vi "LVClass_WavefrontCorrector ctor.vi"(0 "WavefrontCorrector (const)":refnum<class "WavefrontCorrector.lvclass">, 5 "PathToWavefrontCorrectorSetupFile":path, 7 "init_state_from_config_file":bool, 11 "error in (no error)":errorcluster) -> (4 "WavefrontCorrector (new)":refnum<class "WavefrontCorrector.lvclass">, 15 "error out":errorcluster)   [LabVIEW 2020, in "WavefrontCorrector.lvclass"]
doc: "WavefrontCorrector constructor.\n\n--------------------------------------------------------------------------------\n\n<B>correctorIn </B> : Constant Pointer to WavefrontCorrector object.\n<B>correctorOut </B> : Constant Pointer to WavefrontCorrector object.\n<B>config_file_path </B> : Absolute path to Wavefront corrector configuration file.\n<B>ErrorIn </B> : Error\n<B>ErrorOut </B> : Error\n\n--------------------------------------------------------------------------------"
uses:
  WavefrontCorrector.lvclass
  WavefrontCorrectorSet.lvclass
  Wavefront Corrector states - ONE.ctl
  WavefrontCorrector.lvclass/WavefrontCorrector.ctl
  Handle creation.ctl
  LVClass_WavefrontCorrectorSet Read AllWavefrontCorrectorParametersProperties.vi
  LVClass_WavefrontCorrectorSet Read AllValueSetAndGet.vi
  LVClass_WavefrontCorrectorSet Read AllValueGet.vi
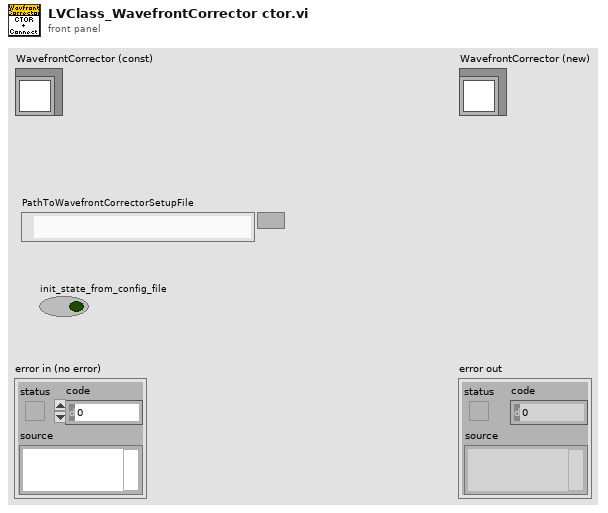
[diagram p1: front panel]
types:
  T1 = typedef "Wavefront Corrector states - ONE.ctl" = cluster{"Max":sgl, "Min":sgl, "Validity":enum16{"valid", "fixed", "invalid"}, "Fixed_Position":sgl}
  T2 = typedef "Handle creation.ctl" = enum16{"By ctor", "By write function"}
  T3 = typedef "WavefrontCorrectorSpecifications.ctl" = cluster{"Mirror name":string, "Plugin name":string, "Serial number":string, "Revision":string, "Number of commands":i32, "Sleep after command apply (ms)":i32, "Has internal memory ?":bool}
  T4 = typedef "ParameterID.ctl" = cluster{"Name":string, "ConnectionParameter?":bool, "Type":T5, "Authorization":T6, "OnFlyAuthorization":T7, "StringValue":string, "Value":dbl, "Min":dbl, "Max":dbl, "BooleanValue":bool, "StringParameterList":string[]}
  T5 = typedef "CameraParameters_Type.ctl" = enum16{"Integer", "Real", "String", "Boolean"}
  T6 = typedef "CameraParameters_Authorization.ctl" = enum16{"Disable", "Gettable", "Settable - Gettable"}
  T7 = typedef "CameraParameters_OnFlyAuthorization.ctl" = enum16{"None", "Gettable", "Settable", "Settable - Gettable"}
  T8 = typedef "CameraParametersSetup.ctl" = cluster{"Name":string, "Type":T5, "Value":dbl, "BooleanValue":bool, "StringValue":string, "ConnectionParameter":bool}
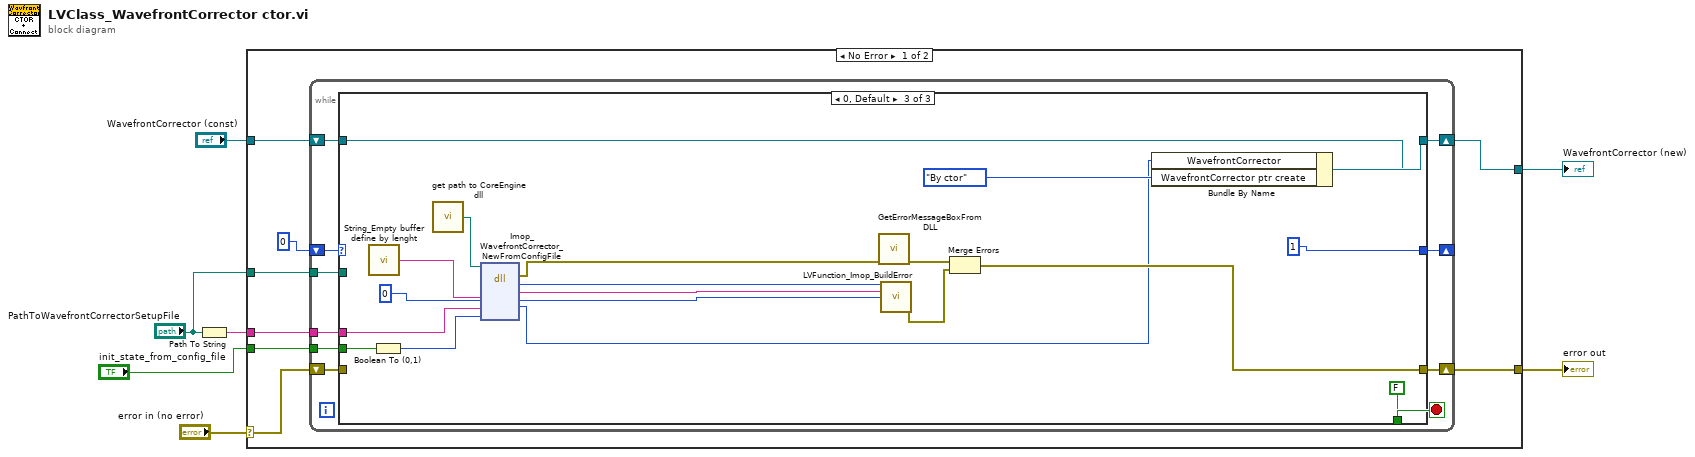
[diagram p0: block diagram]
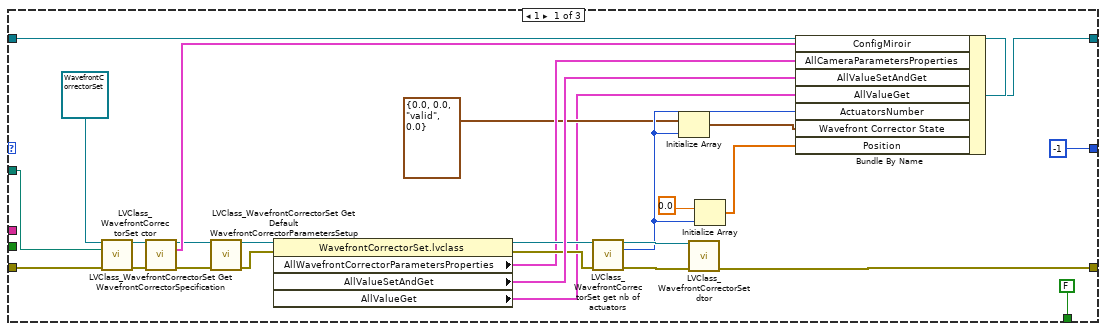
[diagram p2: hidden frame]
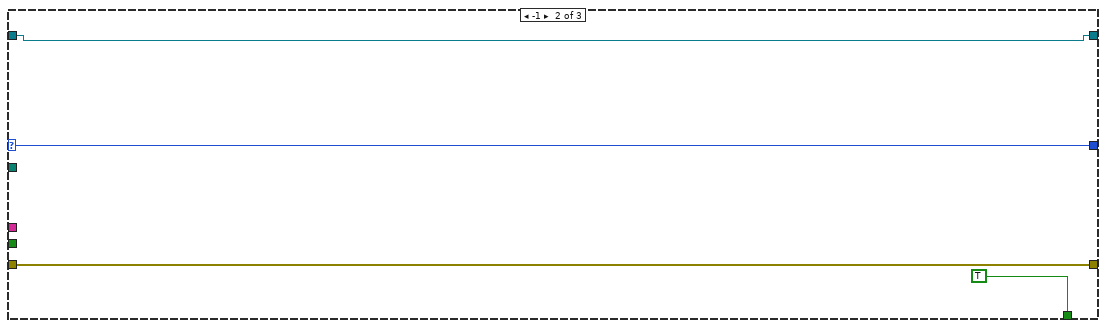
[diagram p3: hidden frame]
diagram:
  n1 = Path To String(path="PathToWavefrontCorrectorSetupFile") -> (string=w7:string)
  n2 = case shown="No Error" "error in (no error)" {
    selector: "error in (no error)" -> [w10 w76]
    tunnel: [w9 w76] -> w4
    tunnel: [w14 w75] -> w3
    tunnel: "WavefrontCorrector (const)" -> [w15 w75]
    tunnel: w7 -> [w13 _]
    tunnel: "PathToWavefrontCorrectorSetupFile" -> [w11 _]
    tunnel: "init_state_from_config_file" -> [w8 _]
    frame No Error {
      n3 = while {
        tunnel: w13 -> [w24]
        shift-right: [w22] -> _
        shift-left: 0 -> [w23]
        tunnel: w11 -> [w21]
        shift-right: [w18] -> w9
        shift-left: w10 -> [w19]
        shift-right: [w25] -> w14
        shift-left: w15 -> [w20]
        tunnel: w8 -> [w16]
        stop <- w17 stop-if-true
        n4 = case shown="0, Default" w23 {
          selector: w23 -> [_ w56 _]
          tunnel: [w40 w53 w68] -> w25
          tunnel: [w41 w55 w65] -> w18
          tunnel: w24 -> [_ _ w64]
          tunnel: [-1 w56 1] -> w22
          tunnel: w21 -> [w50 _ _]
          tunnel: w20 -> [w49 w53 w61]
          tunnel: w19 -> [w46 w55 _]
          tunnel: [FALSE TRUE FALSE] -> w17
          tunnel: w16 -> [_ _ w59]
          frame 1 {
            n5 = call "LVClass_WavefrontCorrectorSet ctor.vi"("WavefrontCorrectorSet (const)"=refnum<class "WavefrontCorrectorSet.lvclass"> refnum ("WavefrontCorrectorSet.lvclass"), "PathToWavefrontCorrectorSetupFile"=w50, "error in (no error)"=w46) -> ("WavefrontCorrectorSet (new)"=w52:refnum<class "WavefrontCorrectorSet.lvclass">, "error out"=w47:errorcluster)  [unwired: 11 in]
            n6 = call "LVClass_WavefrontCorrectorSet Get WavefrontCorrectorSpecification.vi"("WavefrontCorrectorSet in"=w52, "error in (no error)"=w47) -> ("WavefrontCorrectorSet out"=w34:refnum<class "WavefrontCorrectorSet.lvclass">, "ConfigMiroir"=w48:T3, "error out"=w35:errorcluster)  [unwired: 11 in]
            n7 = call "LVClass_WavefrontCorrectorSet Get Default WavefrontCorrectorParametersSetup.vi"("WavefrontCorrectorSet in"=w34, "error in (no error)"=w35) -> ("WavefrontCorrectorSet out"=w32:refnum<class "WavefrontCorrectorSet.lvclass">, "error out"=w30:errorcluster)  [unwired: 9 in, 3 out]
            n8 = property class="WavefrontCorrectorSet.lvclass"(reference=w32, error in=w30) -> (reference out=w31:refnum<class "WavefrontCorrectorSet.lvclass">, error out=w29:errorcluster, "AllWavefrontCorrectorParametersProperties"=w28:T4[], "AllValueSetAndGet"=w33:T8[], "AllValueGet"=w26:T8[])
            n9 = call "LVClass_WavefrontCorrectorSet get nb of actuators.vi"("WavefrontCorrectorSet in"=w31, "error in (no error)"=w29) -> ("WavefrontCorrectorSet out"=w43:refnum<class "WavefrontCorrectorSet.lvclass">, "ActuatorsNumber"=w37:i32, "error out"=w42:errorcluster)  [unwired: 11 in]
            n10 = Initialize Array(T1 {"Max"=0.0, "Min"=0.0, "Validity"=enum."valid", "Fixed_Position"=0.0} ("Actuator State"), w37) -> (w39:T1[])
            n11 = call "LVClass_WavefrontCorrectorSet dtor.vi"("WavefrontCorrectorSet in"=w43, "error in (no error)"=w42) -> ("error out"=w41:errorcluster)  [unwired: 12 in, 1 out]
            n12 = Initialize Array(sgl 0.0 ("Numeric"), w37) -> (w36:sgl[])
            n13 = Bundle By Name(cluster=w49, "ConfigMiroir"=w48, "AllCameraParametersProperties"=w28, "AllValueSetAndGet"=w33, "AllValueGet"=w26, "ActuatorsNumber"=w37, "Wavefront Corrector State"=w39, "Position"=w36) -> (w40:refnum<class "WavefrontCorrector.lvclass">)
          }
          frame -1 {
          }
          frame 0, Default {
            n14 = call "String_Empty buffer define by lenght.vi"() -> ("Empty buffer"=w74:string)  [unwired: 1 in]
            n15 = Boolean To (0,1)(Boolean=w59) -> (0, 1=w58:i16)
            n16 = call "get path to CoreEngine dll.vi"() -> ("path to wavekit library"=w71:path)  [unwired: 14 in, 1 out]
            n17 = dll-call lib="D:/soft/HASO_v3/SVN_trunk/ImOpCoreEngine4_LV2011/DLLs/c_interface_vc100.dll" fn="Imop_WavefrontCorrector_NewFromConfigFile"(path in=w71, "message"=w74, "WavefrontCorrector"=0 ("Pupil"), "Config_file_path"=w64, "init_state_from_config_file"=w58) -> (error out=w70:errorcluster, "return type"=w72:i32, "message"=w73:string, "WavefrontCorrector"=w57:i64)  [unwired: 4 in, 1 out]
            n18 = call "GetErrorMessageBoxFromDLL.vi"("error IN"=w70) -> ("error OUT"=w67:errorcluster)  [unwired: 10 in]
            n19 = call "LVFunction_Imop_BuildError.vi"("code"=w72, "String to Prepend to source (\"\")"=w73, "Adresse"=w57) -> ("error out"=w66:errorcluster)  [unwired: 12 in]
            n20 = Merge Errors(w67, w66) -> (w65:errorcluster)
            n21 = Bundle By Name(cluster=w61, "WavefrontCorrector"=w57, "WavefrontCorrector ptr create"=Handle_creation."By ctor" ("Pupil ptr create")) -> (w68:refnum<class "WavefrontCorrector.lvclass">)
          }
        }
      }
    }
    frame Error {
    }
  }
  "error out" <- w4
  "WavefrontCorrector (new)" <- w3
